vi "processTel.vi"(8 "error in (no error)":errorcluster, 10 "packet":string, 11 "TcpServerTel in":refnum<class "TcpServerTel.lvclass">) -> (0 "error out":errorcluster, 3 "TcpServerTel out":refnum<class "TcpServerTel.lvclass">)   [LabVIEW 2018, in "TcpServerTel.lvclass"]
doc: "Process the incoming telemetry. If telemetry is already registered, it will be sent to LabVIEW Component."
uses:
  TcpServerTel/TcpServerTel.lvclass
  home/pcortes/github/ts_labview_tcp_json/src/TcpServerBase/TcpServerBase.lvclass
  TcpServerBase/TcpServerBase.lvclass
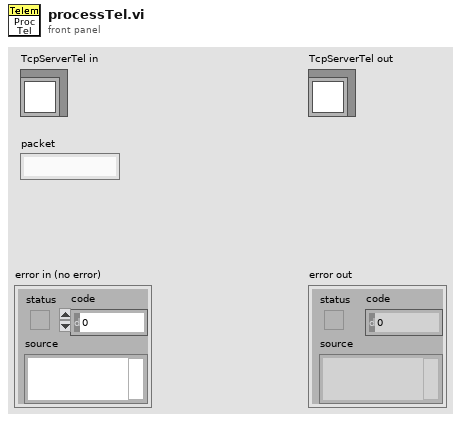
[diagram p1: front panel]
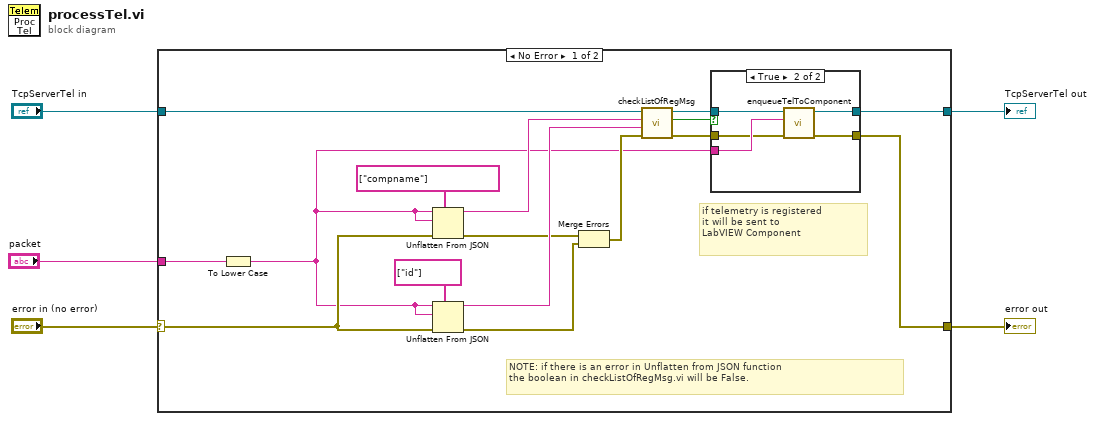
[diagram p0: block diagram]
diagram:
  n1 = case shown="No Error" "error in (no error)" {
    selector: "error in (no error)" -> [w18 w30]
    tunnel: [w8 w30] -> w4
    tunnel: [w14 w29] -> w2
    tunnel: "TcpServerTel in" -> [w20 w29]
    tunnel: "packet" -> [w7 _]
    frame No Error {
      # "if telemetry is registered\nit will be sent to \nLabVIEW Component"
      # "NOTE: if there is an error in Unflatten from JSON function\nthe boolean in checkListOfRegMsg.vi will be False."
      n2 = To Lower Case(string=w7) -> (all lower case string=w6:string)
      n3 = Unflatten From JSON(path=string[] ["compname"] ("tcp packet"), JSON string=w6, type and defaults=w6, error in (no error)=w18) -> (value=w17:string, error out=w11:errorcluster)  [unwired: 3 in]
      n4 = Unflatten From JSON(path=string[] ["id"] ("tcp packet"), JSON string=w6, type and defaults=w6, error in (no error)=w18) -> (value=w16:string, error out=w9:errorcluster)  [unwired: 3 in]
      n5 = Merge Errors(w11, w9) -> (w10:errorcluster)
      n6 = call "checkListOfRegMsg.vi"("error in (no error)"=w10, "msgName"=w16, "compName"=w17, "tcpServerBase in"=w20) -> ("error out"=w13:errorcluster, "msgRegistered?"=w12:bool, "tcpServerBase out"=w15:refnum<class "TcpServerTel.lvclass">)  [unwired: 5 in]
      n7 = case shown="True" w12 {
        tunnel: w15 -> [w23 w26]
        tunnel: [w23 w25] -> w14
        tunnel: w13 -> [w22 w24]
        tunnel: w6 -> [_ w28]
        tunnel: [w22 w27] -> w8
        frame False {
        }
        frame True {
          n8 = call "enqueueTelToComponent.vi"("error in (no error)"=w24, "Elements to enqueue"=w28, "TcpServerTel in"=w26) -> ("error out"=w27:errorcluster, "TcpServerTel out"=w25:refnum<class "TcpServerTel.lvclass">)  [unwired: 7 in]
        }
      }
    }
    frame Error {
    }
  }
  "error out" <- w4
  "TcpServerTel out" <- w2
